vi "Receiver_Example  RxTx - Kopie.vi"() -> ()   [LabVIEW 2022 SP3]
uses:
  <instrlib>/niUSRP/niUSRP Write Tx Data (CDB Cluster).vi
panel:
  out "x .or. y?":bool
  out "Numeric 2":i32
  out "Numeric":i32
  out "size(s)":i32
  out "output byte stream":u8[](array[numeric])
  out "element":u8
  out "Led2":bool
  out "Led1":bool
  in  "Modulation parameter 2":T1
  in  "stop 2":bool
  out "Waveform Graph":cluster{"t0":dbl, "dt":dbl, "Y":dbl[]}(graph)
  out "Frame Duration":dbl format="%#_6p"
  out "error out 2":errorcluster
  out "Bits length":i32
  out "Bits length 2":i32
  in  "String Non Critical Data":string="Critical Dataaaaa\nCritical Dataaaaa\nCritical Dataaaaa\nCritical Dataaaaa\nCritical Dataaaaa"
  in  "String Critical Data":string="Non Critical Data\nNon Critical Data\nNon Critical Data\nNon Critical Data\nNon Critical Data"
  in  "Alpha":dbl=0.05 min=0.0 max=1.0 step=0.05
  out "Frame Duration 2":dbl format="%#_6p"
  in  "New Non Critical Data":string="Critical Dataaaaa\nCritical Dataaaaa\nCritical Dataaaaa\nCritical Dataaaaa\nCritical Dataaaaa"
  in  "New Critical Data":string="Non Critical Data\nNon Critical Data\nNon Critical Data\nNon Critical Data\nNon Critical Data"
  out "AuxString":string
  out "AuxString 2":string
  in  "Previous Button":bool caption="Both Critical and Non Critical\nData must be equal size."
  in  "OFDM 4QAM / 16QAM":bool
  out "USRP CoercedParamters 2":T2={"coerced IQ rate"=100000.0, "coerced carrier frequency"=100000.0, "coerced gain"=0.0} {"coerced gain" format="%#_6f"; "coerced carrier frequency" format="%#_6p"; "coerced IQ rate" format="%#_6p"}
  in  "error in (no error) 2":errorcluster
  in  "USRP ControledParameters 2":T3={"active antenna"="TX1", "gain"=10.0, "carrier frequency"=2400000000.0, "IQ rate"=2000000.0} {"IQ rate" format="%#_6p"; "carrier frequency" format="%#_6p"; "gain" format="%#_6f"}
  in  "device names 2":refnum<k15>="RIO0"
  out "created new?":bool
  out "XY Graph":cdb[](graph)
  out "Modulation parameter":T1
  out "string 2":string
  out "SIG valid?":bool
  out "Frequency offset":dbl
  in  "stop":bool
  out "USRP CoercedParamters":T2={"coerced IQ rate"=100000.0, "coerced carrier frequency"=100000.0, "coerced gain"=0.0} {"coerced gain" format="%#_6f"; "coerced carrier frequency" format="%#_6p"; "coerced IQ rate" format="%#_6p"}
  out "error out":errorcluster
  in  "Trigger level":dbl=0.005 format="%f"
  in  "error in (no error)":errorcluster
  in  "USRP ControledParameters":T3={"active antenna"="RX1", "gain"=10.0, "carrier frequency"=2400000000.0, "IQ rate"=2000000.0} {"IQ rate" format="%#_6p"; "carrier frequency" format="%#_6p"; "gain" format="%#_6f"}
  in  "device names":refnum<k15>="RIO0"
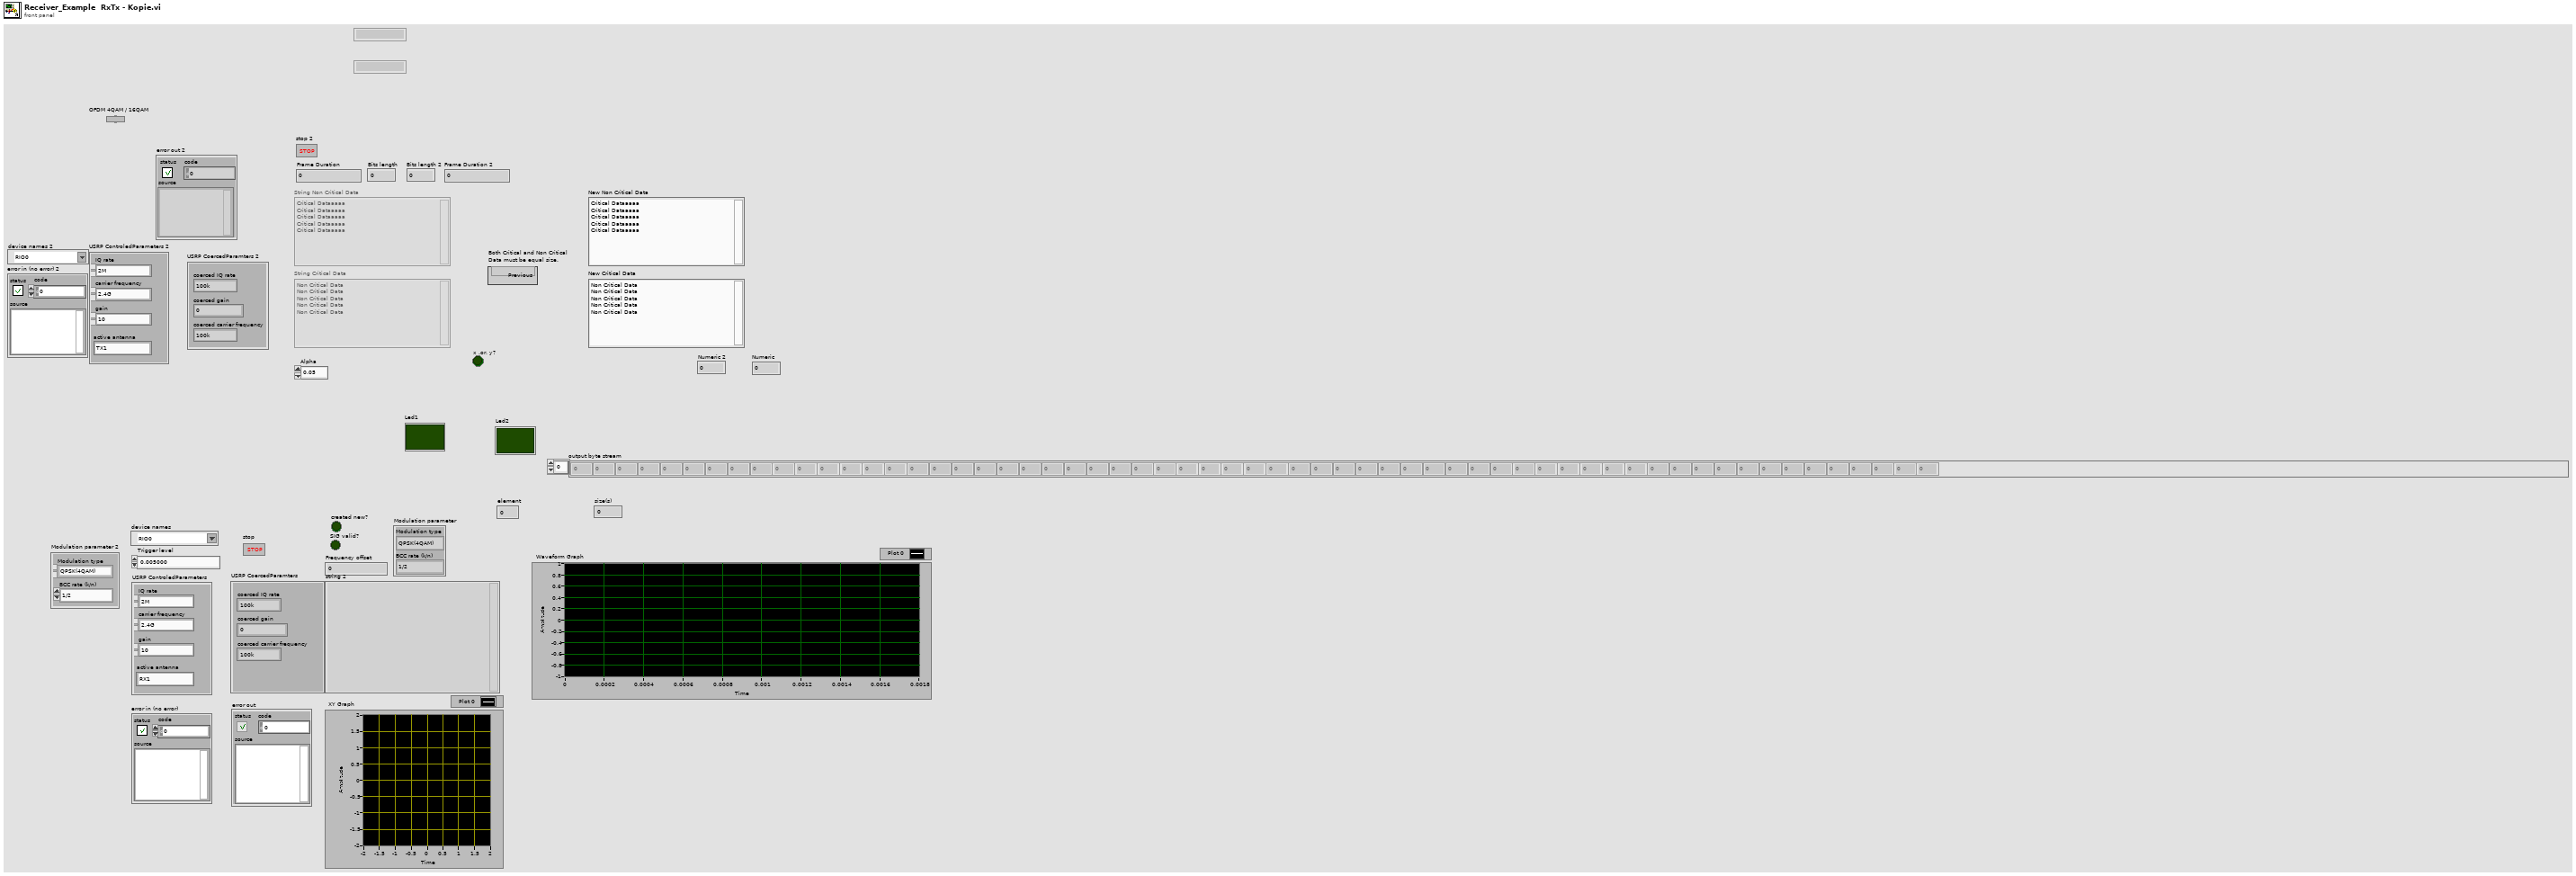
[diagram p1: front panel]
types:
  T1 = cluster{"Modulation type":enum16{"QPSK(4QAM)", "64QAM", "16QAM", "BPSK"}, "BCC rate (k/n)":enum16{"1/2", "2/3", "3/4"}}
  T2 = cluster{"coerced IQ rate":dbl, "coerced carrier frequency":dbl, "coerced gain":dbl}
  T3 = cluster{"active antenna":string, "gain":dbl, "carrier frequency":dbl, "IQ rate":dbl}
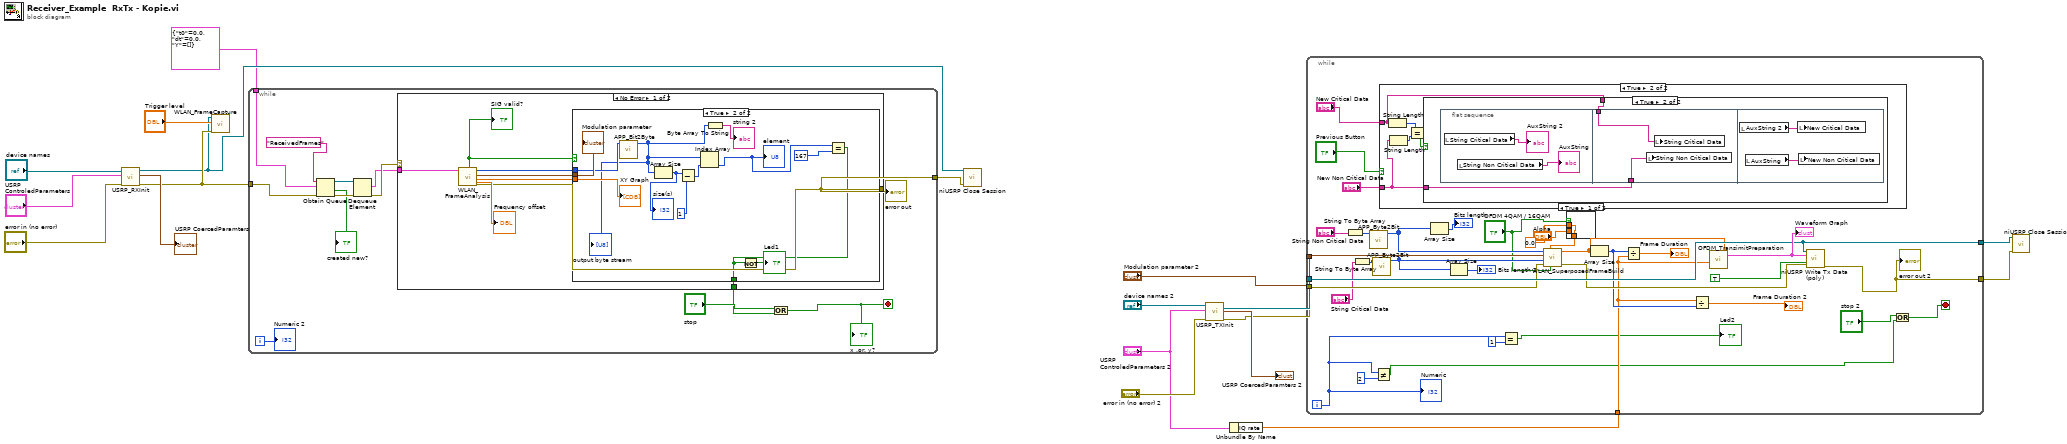
[diagram p0: block diagram]
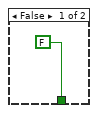
[diagram p5: hidden frame]
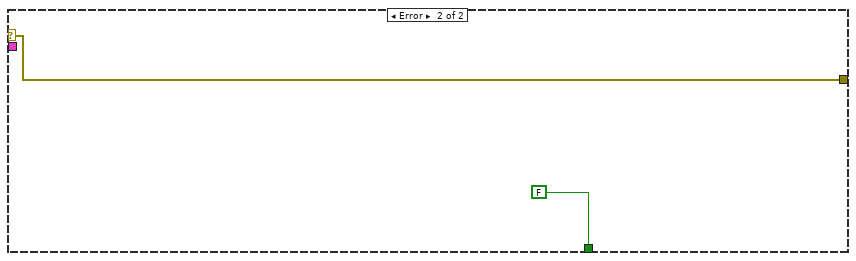
[diagram p6: hidden frame]
diagram:
  n1 = call "USRP_RXInit.vi"("device names"="device names", "USRP ControledParameters"="USRP ControledParameters", "error in (no error)"="error in (no error)") -> ("session handle out"=w12:refnum<k15>, "USRP CoercedParamters"=→"USRP CoercedParamters":T2, "error out"=w15:errorcluster)  [unwired: 5 in]
  n2 = call "WLAN_FrameCapture.vi"("error in (no error)"=w15, "Trigger level"="Trigger level", "session handle"=w12) -> ()  [unwired: 8 in]
  n3 = while {
    tunnel: w15 -> [w31]
    tunnel: cluster{"t0":dbl, "dt":dbl, "Y":cdb[]} {"t0"=0.0, "dt"=0.0, "Y"=[]} ("data") -> [w32]
    tunnel: [w24] -> w13
    i -> [w20]
    stop <- w22 stop-if-true
    n4 = Obtain Queue(name (unnamed)="ReceivedFrames", element data type=w32, error in (no error)=w31) -> (queue out=w30:refnum<queue>, created new?=→"created new?":bool, error out=w27:errorcluster)  [unwired: 2 in]
    n5 = Dequeue Element(queue=w30, error in (no error)=w27) -> (element=w28:cluster{"t0":dbl, "dt":dbl, "Y":cdb[]}, error out=w29:errorcluster)  [unwired: 1 in, 2 out]
    n6 = case shown="No Error" w29 {
      selector: w29 -> [_ w55]
      tunnel: w28 -> [w34 _]
      tunnel: [w35 w55] -> w24
      tunnel: [w33 FALSE] -> w21
      frame No Error {
        n7 = call "WLAN_FrameAnalysis.vi"("input cluster"=w34) -> ("error out"=w35:errorcluster, "Constellation"=w37:cdb[], "Modulation parameter"=w36:T1, "output bits"=w38:i8[], "Frequency offset"=→"Frequency offset":dbl, "SIG valid?"=w39:bool)  [unwired: 5 in]
        "SIG valid?" <- w39
        n8 = case shown="True" w39 {
          tunnel: w38 -> [_ w50]
          tunnel: w37 -> [_ w52]
          tunnel: w36 -> [_ w53]
          tunnel: [FALSE w42] -> w33
          frame False {
          }
          frame True {
            n9 = call "APP_Bit2Byte.vi"("input bit stream"=w50) -> ("output byte stream"=w49:u8[])  [unwired: 10 in]
            "output byte stream" <- w49
            n10 = Array Size(array=w49) -> (size(s)=w47:i32)
            "size(s)" <- w47
            n11 = Subtract(x=w47, y=1) -> (x-y=w46:i32)
            n12 = Index Array(array=w49, index=w46) -> (element=w44:u8)
            "element" <- w44
            n13 = Byte Array To String(unsigned byte array=w49) -> (string=→"string 2":string)
            n14 = Equal?(x=w44, y=u8 167) -> (x = y?=w42:bool)
            n15 = Not(x=w42) -> (.not. x?=→"Led1":bool)
            "Modulation parameter" <- w53
            "XY Graph" <- w52
          }
        }
      }
      frame Error {
      }
    }
    "error out" <- w24
    n16 = Or(x="stop", y=w21) -> (x .or. y?=w22:bool)
    "x .or. y?" <- w22
    "Numeric 2" <- w20
  }
  n17 = call <instrlib>:"niUSRP Close Session.vi"("session handle"=w12, "error in (no error)"=w13) -> ()  [unwired: 13 in, 1 out]
  n18 = call "USRP_TXInit.vi"("device names"="device names 2", "USRP ControledParameters"="USRP ControledParameters 2", "error in (no error)"="error in (no error) 2") -> ("session handle out"=w8:refnum<k15>, "USRP CoercedParamters"=→"USRP CoercedParamters 2":T2, "error out"=w4:errorcluster)  [unwired: 5 in]
  n19 = Unbundle By Name("USRP ControledParameters 2") -> ("IQ rate"=w1:dbl)
  n20 = while {
    tunnel: w8 -> [w85]
    tunnel: "Modulation parameter 2" -> [w79]
    tunnel: w4 -> [w78]
    tunnel: w1 -> [w73]
    tunnel: [w85] -> w3
    tunnel: [w84] -> w2
    i -> [w57]
    stop <- w62 stop-if-true
    n21 = String To Byte Array(string="String Non Critical Data") -> (unsigned byte array=w82:u8[])
    n22 = String To Byte Array(string="String Critical Data") -> (unsigned byte array=w81:u8[])
    n23 = call "APP_Byte2Bit.vi"("input byte stream"=w82) -> ("output bit stream"=w75:i8[])  [unwired: 10 in]
    n24 = call "APP_Byte2Bit.vi"("input byte stream"=w81) -> ("output bit stream"=w80:i8[])  [unwired: 10 in]
    n25 = Not Equal?(x=w57, y=2) -> (x != y?=w56:bool)
    n26 = case shown="True" "Previous Button" {
      tunnel: "New Non Critical Data" -> [_ w96]
      tunnel: "New Critical Data" -> [_ w92]
      frame False {
      }
      frame True {
        n27 = String Length(string=w92) -> (length=w95:i32)
        n28 = String Length(string=w96) -> (length=w94:i32)
        n29 = Equal?(x=w95, y=w94) -> (x = y?=w93:bool)
        n30 = case shown="True" w93 {
          tunnel: w96 -> [_ w98]
          tunnel: w92 -> [_ w97]
          frame False {
          }
          frame True {
            n31 = flat-sequence {
              tunnel: w98 -> [w102]
              tunnel: w97 -> [w101]
              frame #0 {
                n32 = local read "String Critical Data"() -> (→"AuxString 2":string)
                n33 = local read "String Non Critical Data"() -> (→"AuxString":string)
              }
              frame #1 {
                n34 = local write "String Non Critical Data"(w102) -> ()
                n35 = local write "String Critical Data"(w101) -> ()
              }
              frame #2 {
                n36 = local read "AuxString 2"() -> (w103:string)
                n37 = local read "AuxString"() -> (w104:string)
                n38 = local write "New Critical Data"(w103) -> ()
                n39 = local write "New Non Critical Data"(w104) -> ()
              }
            }
          }
        }
      }
    }
    n40 = Array Size(array=w75) -> (size(s)=→"Bits length":i32)
    n41 = Array Size(array=w80) -> (size(s)=→"Bits length 2":i32)
    n42 = Equal?(x=w57, y=1) -> (x = y?=→"Led2":bool)
    n43 = case shown="True" "OFDM 4QAM / 16QAM" {
      tunnel: [w90 w91] -> w67
      tunnel: "Alpha" -> [_ w91]
      tunnel: 0.0 ("Alpha 2") -> [w90 _]
      frame True {
      }
      frame False {
      }
    }
    n44 = call "WLAN_SuperposedFrameBuild.vi"("OFDMON"="OFDM 4QAM / 16QAM", "Alpha"=w67, "error in (no error)"=w78, "data in 2"=w80, "Modulation parameter"=w79, "data in"=w75) -> ("error out"=w77:errorcluster, "output array"=w76:cdb[])  [unwired: 4 in]
    n45 = Array Size(array=w76) -> (size(s)=w74:i32)
    n46 = Divide(x=w74, y=w73) -> (x/y=→"Frame Duration":dbl)
    n47 = Divide(x=w73, y=w74) -> (x/y=→"Frame Duration 2":dbl)
    n48 = call "OFDM_TransimitPreparation.vi"("IQ rate"=w73, "array"=w76) -> ("output cluster"=w87:cluster{"t0":dbl, "dt":dbl, "Y":cdb[]})  [unwired: 9 in]
    "Waveform Graph" <- w87
    n49 = call-poly <instrlib>:"niUSRP Write Tx Data (poly).vi"("session handle"=w85, "data"=w87, "end of data?"=TRUE, "error in (no error)"=w77) -> ("error out"=w84:errorcluster)  [unwired: 10 in, 1 out]
    "error out 2" <- w84
    n50 = Or(x="stop 2", y=w56) -> (x .or. y?=w62:bool)
    "Numeric" <- w57
  }
  n51 = call <instrlib>:"niUSRP Close Session.vi"("session handle"=w3, "error in (no error)"=w2) -> ()  [unwired: 13 in, 1 out]
